vi "tof.vi"(8 "Digital in":refnum<vi>, 10 "Time":i32, 11 "START in":bool) -> (2 "ET 4":i32, 3 "Q 4":bool)   [LabVIEW 2020]
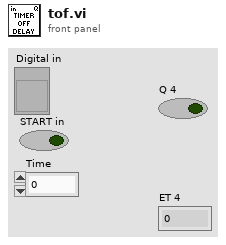
[diagram p1: front panel]
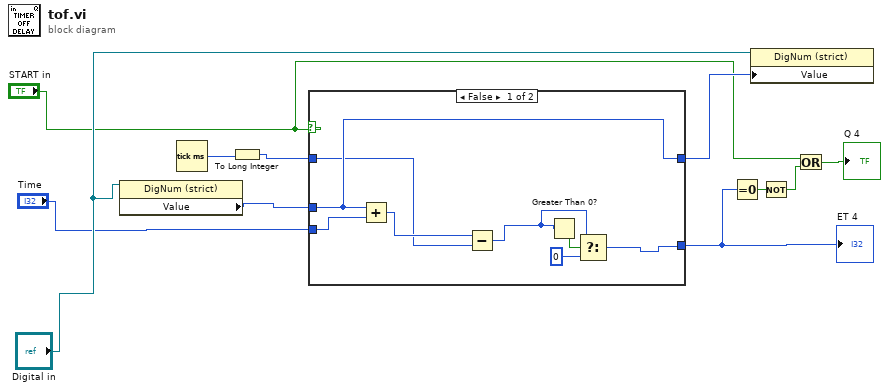
[diagram p0: block diagram]
diagram:
  n1 = property class="DigNum (strict)"(reference="Digital in") -> ("Value"=w8:i32)  [unwired: 1 in, 2 out]
  n2 = Tick Count (ms)() -> (millisecond timer value=w5:u32)
  n3 = To Long Integer(number=w5) -> (32bit integer=w6:i32)
  n4 = case shown="False" "START in" {
    tunnel: w6 -> [w13 w21]
    tunnel: [w14 w21] -> w9
    tunnel: w8 -> [w14 _]
    tunnel: "Time" -> [w15 w20]
    tunnel: [w12 w20] -> w7
    frame False {
      n5 = Add(x=w14, y=w15) -> (x+y=w19:i32)
      n6 = Subtract(x=w19, y=w13) -> (x-y=w17:i32)
      n7 = Greater Than 0?(x=w17) -> (x > 0?=w18:bool)
      n8 = Select(t=w17, s=w18, f=0) -> (s? t:f=w12:i32)
    }
    frame True {
    }
  }
  "ET 4" <- w7
  n9 = Equal To 0?(x=w7) -> (x = 0?=w10:bool)
  n10 = property class="DigNum (strict)"(reference="Digital in", "Value"=w9) -> ()  [unwired: 1 in, 2 out]
  n11 = Not(x=w10) -> (.not. x?=w11:bool)
  n12 = Or(x="START in", y=w11) -> (x .or. y?=→"Q 4":bool)
